vi "Initiate assembly.vi"(8 "error in (no error)":errorcluster, 11 "Database Entry in":refnum<class "Database Entry.lvclass">) -> (0 "error out":errorcluster, 1 "Selected postitions":dbl[](array[numeric]), 2 "Module?":bool, 3 "Database Entry out":refnum<class "Database Entry.lvclass">, 4 "Baselayer Thickness":dbl[](array[numeric]))   [LabVIEW 2021, in "Database Entry.lvclass"]
uses:
  Database Entry.lvclass
  Database Entry.lvclass/Database Entry.ctl
  Stack/Stack.lvclass
panel:
  in  "Type":bool
  out "Status":dbl[][](array[numeric])
  in  "Operator":u16(ring)
  in  "Assembly Region":T1
  in  "Submit":bool
  in  "Geometry":u16(ring) items=["Full", "Top", "Bottom", "Left", "Right", "Five"]
  in  "Resolution":u16(ring) items=["LD", "HD"]
  # "Protomodule"
  # "Module"
  # "Tray Slot 1"
  # "Slot 2"
  # "Slot 3"
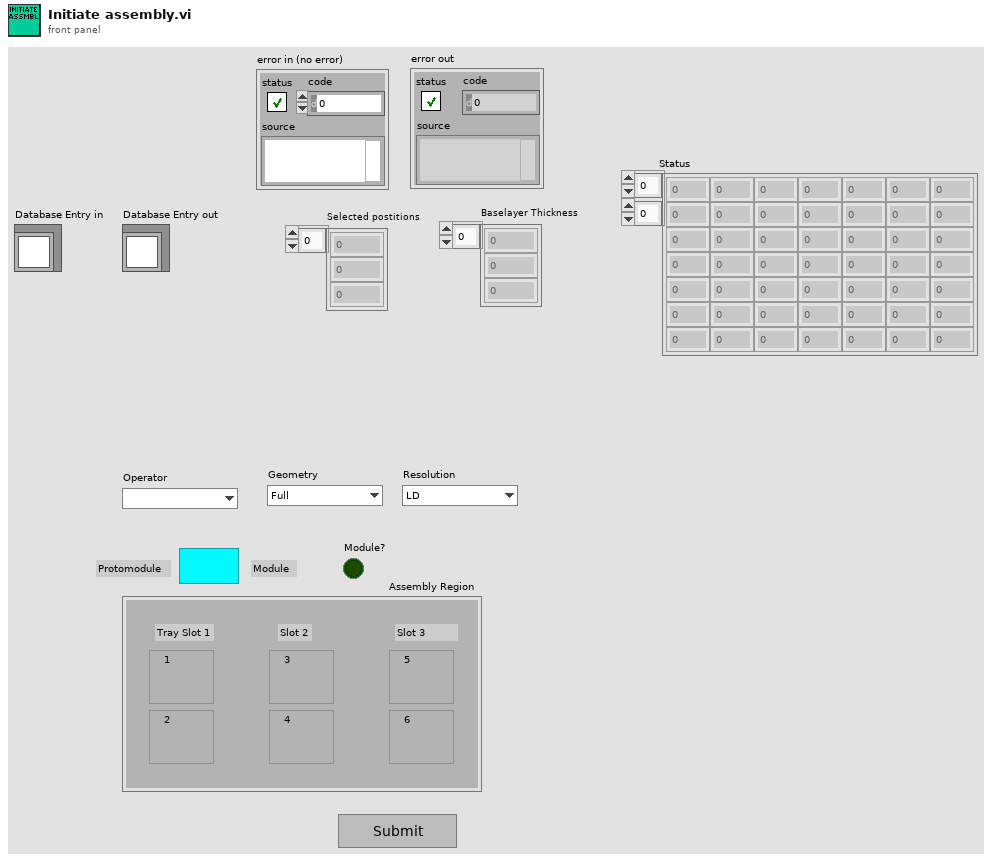
[diagram p1: front panel]
types:
  T1 = cluster{"1":bool, "2":bool, "3":bool, "4":bool, "5":bool, "6":bool}
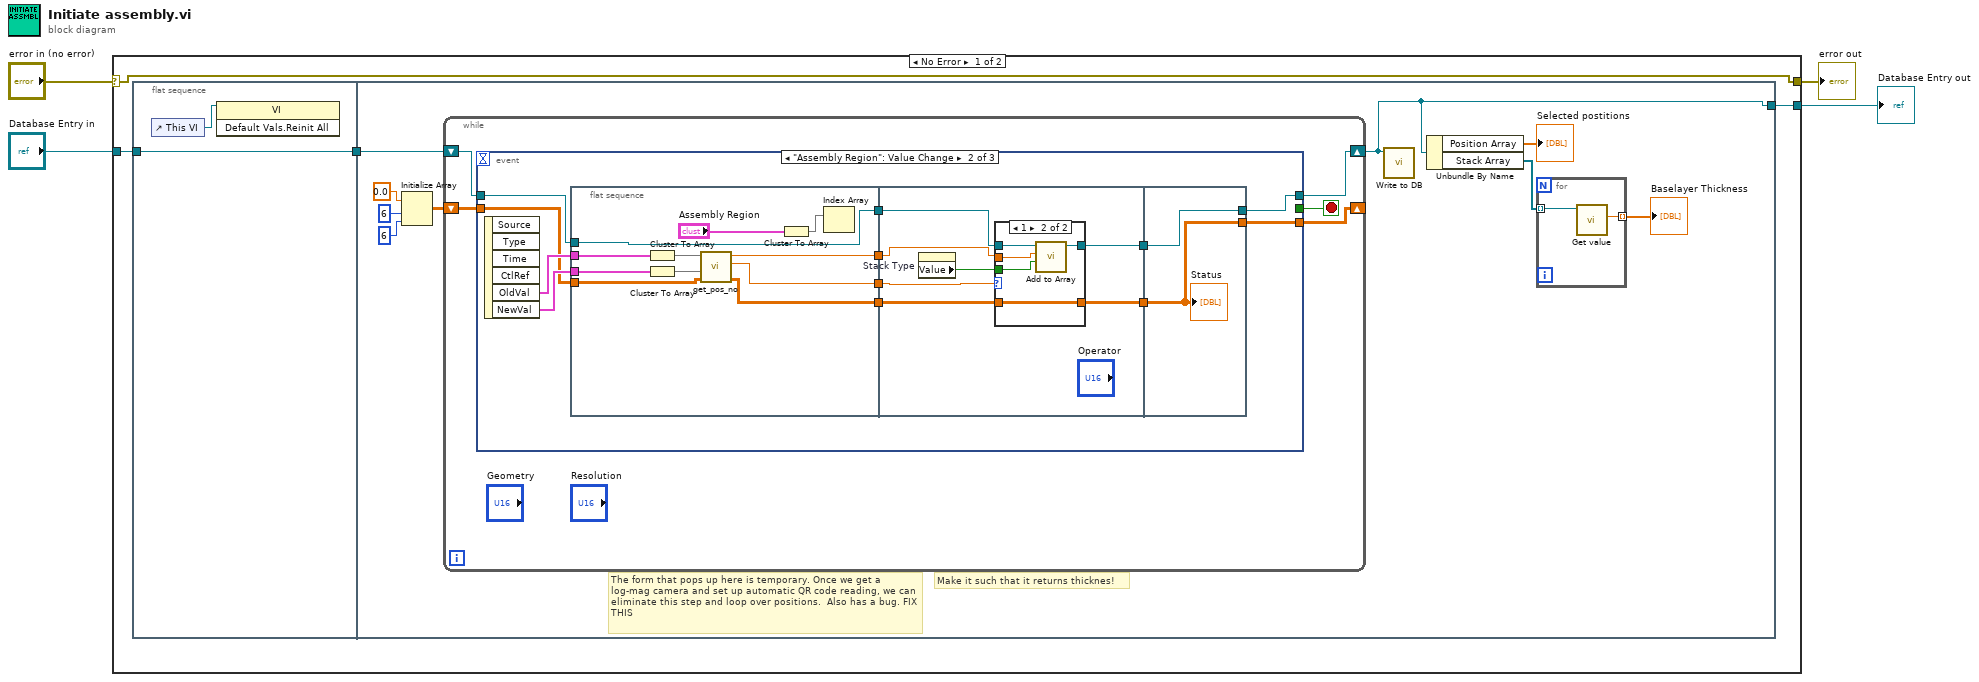
[diagram p0: block diagram]
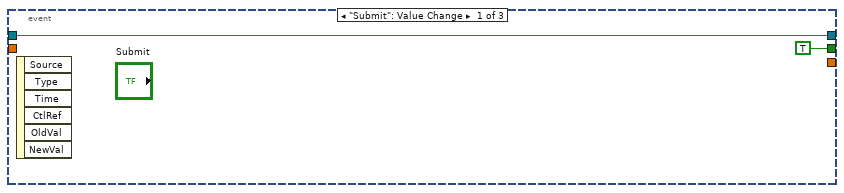
[diagram p2: hidden frame]
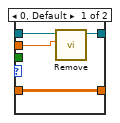
[diagram p3: hidden frame]
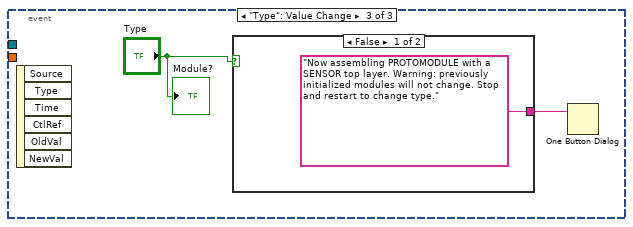
[diagram p4: hidden frame]
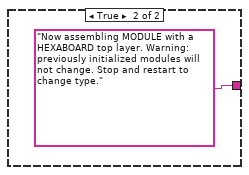
[diagram p5: hidden frame]
diagram:
  n1 = case shown="No Error" "error in (no error)" {
    selector: "error in (no error)" -> [w8 w75]
    tunnel: [w8 w75] -> w3
    tunnel: [w6 w74] -> w1
    tunnel: "Database Entry in" -> [w7 w74]
    frame No Error {
      n2 = flat-sequence {
        tunnel: w7 -> [w10]
        tunnel: [w10] -> w5
        tunnel: [w14] -> w6
        tunnel: w5 -> [w19]
        frame #0 {
          n3 = control-ref of="This VI"() -> (w9:refnum<vi>)
          n4 = invoke class="VI" method="Default Vals.Reinit All"(reference=w9) -> ()  [unwired: 2 in, 3 out]
        }
        frame #1 {
          # "The form that pops up here is temporary. Once we get a log-mag camera and set up automatic QR code reading, we can eliminate this step and loop over positions.  Also has a bug. FIX THIS"
          # "Make it such that it returns thicknes!"
          n5 = Initialize Array(0.0 ("element"), 6 ("dimension size"), 6 ("dimension size")) -> (w18:dbl[][])
          n6 = while {
            shift-right: [w25] -> w14
            shift-left: w19 -> [w22]
            shift-right: [w23] -> _
            shift-left: w18 -> [w24]
            stop <- w26 stop-if-true
            n7 = event shown="[1] \"Assembly Region\": Value Change" {
              selector: _ -> [_ _ _]
              dyn-events: _ -> [_ _ _]
              timeout: _ -> [_ _ _]
              tunnel: [TRUE _ _] -> w26
              tunnel: w22 -> [w27 w33 _]
              tunnel: [w27 w30 _] -> w25
              tunnel: w24 -> [_ w38 _]
              tunnel: [_ w34 _] -> w23
              event "Submit": Value Change {
                n8 = event-data() -> ()  [unwired: 1 in, 6 out]
              }
              event "Assembly Region": Value Change {
                n9 = event-data() -> ("OldVal"=w39:T1, "NewVal"=w40:T1)  [unwired: 1 in, 4 out]
                n10 = flat-sequence {
                  tunnel: w40 -> [w50]
                  tunnel: w39 -> [w49]
                  tunnel: w38 -> [w45]
                  tunnel: [w42] -> w36
                  tunnel: [w44] -> w35
                  tunnel: w33 -> [w43]
                  tunnel: [w43] -> w32
                  tunnel: [w41] -> w31
                  tunnel: [w57] -> w37
                  tunnel: w36 -> [w58]
                  tunnel: w35 -> [w55]
                  tunnel: w32 -> [w56]
                  tunnel: w31 -> [w54]
                  tunnel: [w53] -> w29
                  tunnel: w37 -> [w69]
                  tunnel: [w69] -> w34
                  tunnel: [w68] -> w30
                  tunnel: w29 -> [w68]
                  frame #0 {
                    n11 = Cluster To Array(cluster=w49) -> (array=w46:bool[])
                    n12 = Cluster To Array(cluster=w50) -> (array=w47:bool[])
                    n13 = call "get_pos_no.vi"("Status Old"=w45, "Array New Status"=w47, "Array Old Status"=w46) -> ("Status New"=w42:dbl[][], "State"=w41:dbl, "Position ID"=w44:dbl)  [unwired: 2 in]
                    n14 = Cluster To Array(cluster="Assembly Region") -> (array=w51:bool[])
                    n15 = Index Array(array=w51) -> ()  [unwired: 1 in, 1 out]
                  }
                  frame #1 {
                    n16 = property on="Stack Type" class="Bool (strict)"() -> ("Value"=w52:bool)  [unwired: 2 in, 2 out]
                    n17 = case shown="1" w54 {
                      tunnel: w58 -> [w59 w67]
                      tunnel: [w59 w67] -> w57
                      tunnel: w56 -> [w62 w66]
                      tunnel: [w61 w65] -> w53
                      tunnel: w55 -> [w60 w64]
                      tunnel: w52 -> [_ w63]
                      frame 0, Default {
                        n18 = call "Remove.vi"("Index"=w60, "Database Entry in"=w62) -> ("Database Entry out"=w61:refnum<class "Database Entry.lvclass">)  [unwired: 8 in, 1 out]
                      }
                      frame 1 {
                        n19 = call "Add to Array.vi"("Module?"=w63, "Position Index"=w64, "Database Entry in"=w66) -> ("Database Entry out"=w65:refnum<class "Database Entry.lvclass">)  [unwired: 7 in, 1 out]
                      }
                    }
                  }
                  frame #2 {
                    "Status" <- w69
                  }
                }
              }
              event "Type": Value Change {
                n20 = event-data() -> ()  [unwired: 1 in, 6 out]
                n21 = case shown="False" "Type" {
                  tunnel: ["Now assembling PROTOMODULE with a SENSOR top layer. Warning: previously initialized modules will not change. Stop and restart to change type." "Now assembling MODULE with a HEXABOARD top layer. Warning: previously initialized modules will not change. Stop and restart to change type."] -> w71
                  frame False {
                  }
                  frame True {
                  }
                }
                n22 = One Button Dialog(message=w71) -> ()  [unwired: 1 in, 1 out]
                "Module?" <- "Type"
              }
            }
          }
          n23 = call "Write to DB.vi"("Database Entry in"=w14) -> ()  [unwired: 9 in, 2 out]
          n24 = Unbundle By Name(w14) -> ("Position Array"=→"Selected postitions":dbl[], "Stack Array"=w12:refnum<class "Stack.lvclass">[])
          n25 = for {
            tunnel: w12 -> [w21] mode=indexing
            tunnel: [w20] -> w11 mode=indexing
            n26 = call "Get value.vi"("Stack in"=w21) -> ("Value"=w20:dbl)  [unwired: 8 in, 2 out]
          }
          "Baselayer Thickness" <- w11
        }
      }
    }
    frame Error {
    }
  }
  "error out" <- w3
  "Database Entry out" <- w1
